vi "IDS_Freeze_Detector.vi"(6 "IDS actif":bool=TRUE, 8 "Seuil variation":dbl, 9 "Nombre de cycles":dbl=5.0, 10 "RPM":dbl, 11 "STATE":string) -> (3 "Freeze detecte":bool)   [LabVIEW 2022 SP3]
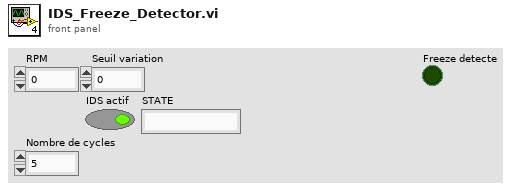
[diagram p1: front panel]
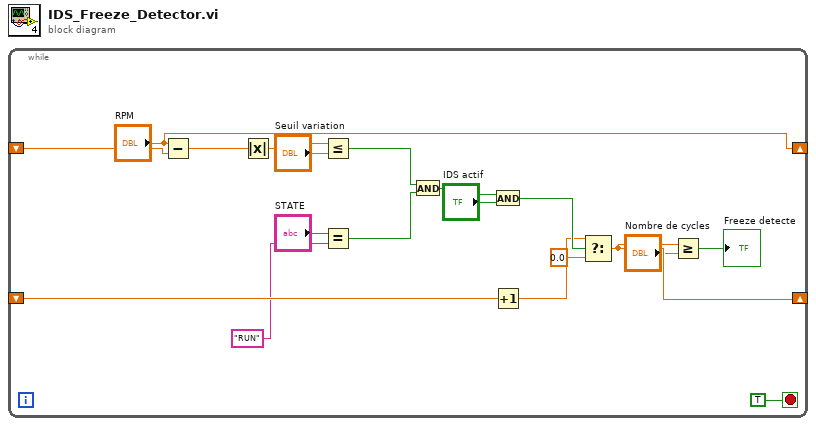
[diagram p0: block diagram]
diagram:
  n1 = while {
    shift-right: ["RPM"] -> _
    shift-left: _ -> [w12]
    shift-right: [w10] -> _
    shift-left: _ -> [w11]
    stop <- TRUE stop-if-true
    n2 = Subtract(x="RPM", y=w12) -> (x-y=w19:dbl)
    n3 = Absolute Value(x=w19) -> (abs(x)=w18:dbl)
    n4 = Less Or Equal?(x=w18, y="Seuil variation") -> (x <= y?=w17:bool)
    n5 = Equal?(x="STATE", y="RUN") -> (x = y?=w16:bool)
    n6 = And(x=w17, y=w16) -> (x .and. y?=w15:bool)
    n7 = And(x=w15, y="IDS actif") -> (x .and. y?=w14:bool)
    n8 = Increment(x=w11) -> (x+1=w13:dbl)
    n9 = Select(t=w13, s=w14, f=0.0) -> (s? t:f=w10:dbl)
    n10 = Greater Or Equal?(x=w10, y="Nombre de cycles") -> (x >= y?=→"Freeze detecte":bool)
  }
